vi "WLAN - Test - UTIL - RxParamaters(DUT).vi"(0 "Rx_Test Parameters":T2 {"OFDM Data Rate (Mbps)" items=["6", "9", "12", "18", "24", "36", "48", "54"]; "DSSS Data Rate (Mbps)" items=["1", "2", "5.5 CCK", "5.5 PBCC", "11 CCK", "11 PBCC", "22", "33"]; "80211n PLCP Frame Format" items=["Mixed Format", "Greenfield Format"]}, 5 "MacAddrSet":string="ALL", 7 "numPackets":i32=200) -> (4 "Rx Paramaters":T1)   [LabVIEW 2011]
uses:
  TV/RW/Includes/WLAN - TV - RW - INC - RxTestParameters.ctl
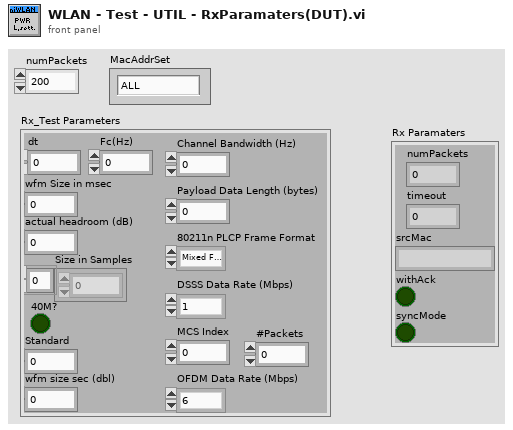
[diagram p1: front panel]
types:
  T1 = cluster{"numPackets":i32, "timeout":i32, "srcMac":string, "withAck":bool, "syncMode":bool}
  T2 = typedef "WLAN - TV - RW - INC - RxTestParameters.ctl" = cluster{"wfm Size in msec":i32, "actual headroom (dB)":dbl, "Size in Samples":i32[], "40M?":bool, "Standard ":i32, "wfm size sec (dbl)":dbl, "dt":dbl, "Channel Bandwidth (Hz)":dbl, "Payload Data Length (bytes)":i32, "80211n PLCP Frame Format":i32, "DSSS Data Rate (Mbps)":i32, "OFDM Data Rate (Mbps)":i32, "MCS Index":i32, "Fc(Hz)":dbl, "#Packets":i32}
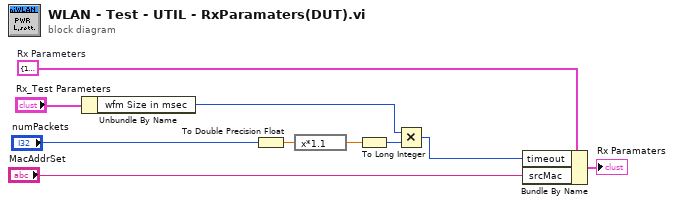
[diagram p0: block diagram]
diagram:
  w6 = T1 {"numPackets"=1000, "timeout"=0, "srcMac"="", "withAck"=FALSE, "syncMode"=FALSE}  # Rx Parameters
  n1 = Unbundle By Name("Rx_Test Parameters") -> ("wfm Size in msec"=w8:i32)
  n2 = To Double Precision Float(number="numPackets") -> (double precision float=w9:dbl)
  n3 = expression code="x*1.1"(w9) -> (w10:dbl)
  n4 = To Long Integer(number=w10) -> (32bit integer=w2:i32)
  n5 = Multiply(x=w8, y=w2) -> (x*y=w4:i32)
  n6 = Bundle By Name(cluster=w6, "timeout"=w4, "srcMac"="MacAddrSet") -> (→"Rx Paramaters":T1)
